vi "Custom Error Popup.vi"(7 "Repeated error?":bool, 8 "VI Error in":errorcluster, 10 "Error to display":errorcluster, 11 "Button Labels":string[](array[string])) -> (0 "error out":errorcluster, 3 "Second Button?":bool)   [LabVIEW 2017]
uses:
  <vilib>/Utility/error.llb/DialogType.ctl
  <vilib>/regexp/Match Regular Expression.xnode
panel:
  in  "Retry":bool
  in  "OK":bool
  in  "System Link Text":bool
  out "Complete call chain:":string
  out "Error Message:":string
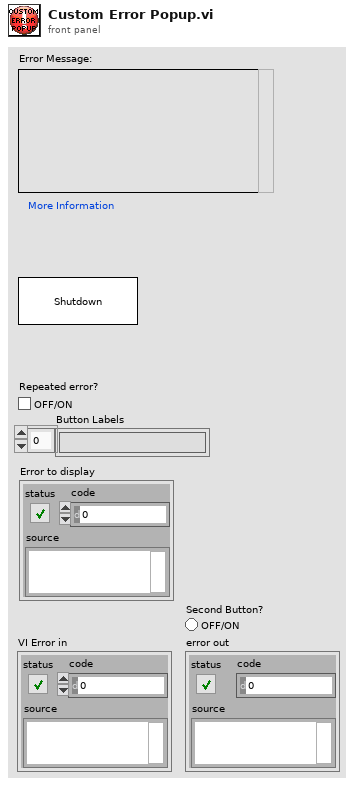
[diagram p1: front panel]
types:
  T1 = enum16{"Always On", "Always Off", "Off While Running"}
  T2 = typedef "DialogType.ctl" = u16
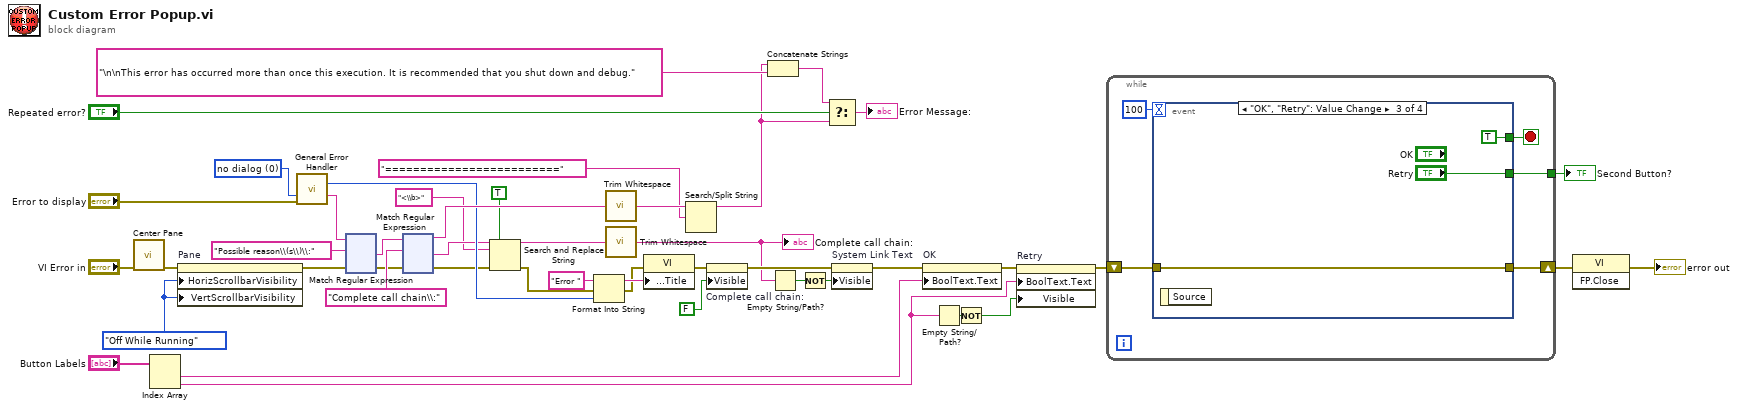
[diagram p0: block diagram]
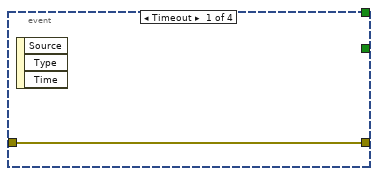
[diagram p2: hidden frame]
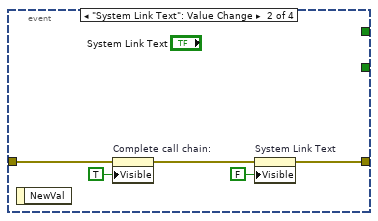
[diagram p3: hidden frame]
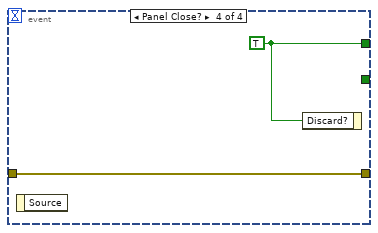
[diagram p4: hidden frame]
diagram:
  w35 = T1."Off While Running" ("Vertical Scrollbar Visibility")
  w46 = T2 0 items=["no dialog", "OK message", "continue or stop message", "OK message + warnings", "continue/stop + warnings"] ("type of dialog (OK msg:1)")
  n1 = call "Center Pane.vi"("error in (no error)"="VI Error in") -> ("error out"=w12:errorcluster)  [unwired: 10 in]
  n2 = Index Array(array="Button Labels") -> (element #1=w21:string, element #2=w20:string)  [unwired: 2 in]
  n3 = property on="Pane" class="Pane"(error in=w12, "HorizScrollbarVisibility"=w35, "VertScrollbarVisibility"=w35) -> (error out=w34:errorcluster)  [unwired: 1 in, 1 out]
  n4 = call <vilib>:"General Error Handler.vi"("type of dialog (OK msg:1)"=w46, "error in (no error)"="Error to display") -> ("code out"=w32:i32, "message"=w45:string)  [unwired: 9 in, 3 out]
  n5 = xnode "Match Regular Expression"("input string"=w45, "regular expression"="Possible reason\\(s\\)\\:", "error in"=w34) -> ("after match"=w43:string, "error out"=w39:errorcluster)  [unwired: 3 in, 3 out]
  n6 = xnode "Match Regular Expression"("input string"=w43, "regular expression"="Complete call chain\\:", "error in"=w39) -> ("before match"=w41:string, "after match"=w5:string, "error out"=w2:errorcluster)  [unwired: 3 in, 2 out]
  n7 = Search and Replace String(replace all?=TRUE ("replace all? (F)"), input string=w5, search string="<\\b>", error in=w2) -> (result string=w6:string, error out=w1:errorcluster)  [unwired: 4 in, 2 out]
  n8 = Format Into String(initial string="Error ", error in=w1, w32) -> (resulting string=w31:string, error out=w30:errorcluster)  [unwired: 1 in]
  n9 = call <vilib>:"Trim Whitespace.vi"("string"=w41) -> ("trimmed string"=w15:string)  [unwired: 1 in]
  n10 = call <vilib>:"Trim Whitespace.vi"("string"=w6) -> ("trimmed string"=w28:string)  [unwired: 1 in]
  "Complete call chain:" <- w28
  n11 = property class="VI"(error in=w30, "Front Panel.Title"=w31) -> (error out=w38:errorcluster)  [unwired: 1 in, 1 out]
  n12 = Search/Split String(string=w15, search string/char (-)="=========================") -> (substring before match=w8:string)  [unwired: 1 in, 2 out]
  n13 = property on="Complete call chain:" class="Str"(error in=w38, "Visible"=FALSE) -> (error out=w37:errorcluster)  [unwired: 1 in, 1 out]
  n14 = Concatenate Strings(w8, "\n\nThis error has occurred more than once this execution. It is recommended that you shut down and debug." ("string")) -> (w7:string)
  n15 = Empty String/Path?(string/path=w28) -> (empty?=w27:bool)
  n16 = Not(x=w27) -> (.not. x?=w26:bool)
  n17 = Select(t=w7, s="Repeated error?", f=w8) -> (s? t:f=→"Error Message:":string)
  n18 = property on="System Link Text" class="Bool"(error in=w37, "Visible"=w26) -> (error out=w17:errorcluster)  [unwired: 1 in, 1 out]
  n19 = property on="OK" class="Bool"(error in=w17, "BoolText.Text"=w21) -> (error out=w23:errorcluster)  [unwired: 1 in, 1 out]
  n20 = Empty String/Path?(string/path=w20) -> (empty?=w19:bool)
  n21 = Not(x=w19) -> (.not. x?=w18:bool)
  n22 = property on="Retry" class="Bool"(error in=w23, "BoolText.Text"=w20, "Visible"=w18) -> (error out=w16:errorcluster)  [unwired: 1 in, 1 out]
  n23 = while {
    shift-right: [w48] -> w25
    shift-left: w16 -> [w49]
    tunnel: [w47] -> w36
    stop <- w50 stop-if-true
    n24 = event shown="[2] \"OK\", \"Retry\": Value Change" {
      selector: _ -> [_ _ _ _]
      dyn-events: _ -> [_ _ _ _]
      timeout: 100 -> [_ _ _ _]
      tunnel: [_ _ TRUE ("System Link Text") w61] -> w50
      tunnel: w49 -> [w52 w55 w60 w62]
      tunnel: [w52 w53 w60 w62] -> w48
      tunnel: [_ _ "Retry" _] -> w47
      event Timeout {
        n25 = event-data() -> ()  [unwired: 1 in, 3 out]
      }
      event "System Link Text": Value Change {
        n26 = event-data() -> ()  [unwired: 1 in, 1 out]
        n27 = property on="Complete call chain:" class="Str"(error in=w55, "Visible"=TRUE) -> (error out=w54:errorcluster)  [unwired: 1 in, 1 out]
        n28 = property on="System Link Text" class="Bool"(error in=w54, "Visible"=FALSE) -> (error out=w53:errorcluster)  [unwired: 1 in, 1 out]
      }
      event "OK", "Retry": Value Change {
        n29 = event-data() -> ()  [unwired: 1 in, 1 out]
      }
      event Panel Close? {
        w61 = TRUE ("System Link Text")
        n30 = event-data() -> ()  [unwired: 1 in, 1 out]
        n31 = event-data("Discard?"=w61) -> ()  [unwired: 1 in, 1 out]
      }
    }
  }
  "Second Button?" <- w36
  n32 = invoke class="VI" method="FP.Close"(error in=w25) -> (error out=→"error out":errorcluster)  [unwired: 2 in, 2 out]
